vi "Position.vi"   [LabVIEW 2011]
uses:
  Robot Global Data.vi
types:
  T1 = typedef "WPI_EncoderDevRef.ctl" = cluster{"DevStatus":errorcluster, "EncoderIndex":T2, "CounterIndex":T3, "DistancePerCount":dbl, "Decoding Type":T4}
  T2 = typedef "FPGA_EncoderIdx.ctl" = enum8{"Enc 0", "Enc 1", "Enc 2", "Enc 3", "Invalid"}
  T3 = typedef "FPGA_CounterCtrSystemIndex.ctl" = enum8{"Ctr 0", "Ctr 1", "Ctr 2", "Ctr 3", "Ctr 4", "Ctr 5", "Ctr 6", "Ctr 7", "Invalid"}
  T4 = typedef "WPI_EncoderType.ctl" = enum16{"1x", "2x", "4x"}
  T5 = typedef "WPI_GyroDevRef.ctl" = cluster{"DevStatus":errorcluster, "Analog Module":T6, "Analog Channel":T7, "Offset":dbl, "Gain (VoltsPerDegree/Second)":dbl}
  T6 = typedef "FPGA_TypedefAnalogModule.ctl" = enum16{"Analog Module 1", "Analog Module 2"}
  T7 = typedef "FPGA_AIChannel.ctl" = enum8{"AI 1", "AI 2", "AI 3", "AI 4", "AI 5", "AI 6", "AI 7", "AI 8", "Invalid"}
  T8 = typedef "Position Typedef.ctl" = cluster{"X":dbl, "Y":dbl, "Heading":dbl}
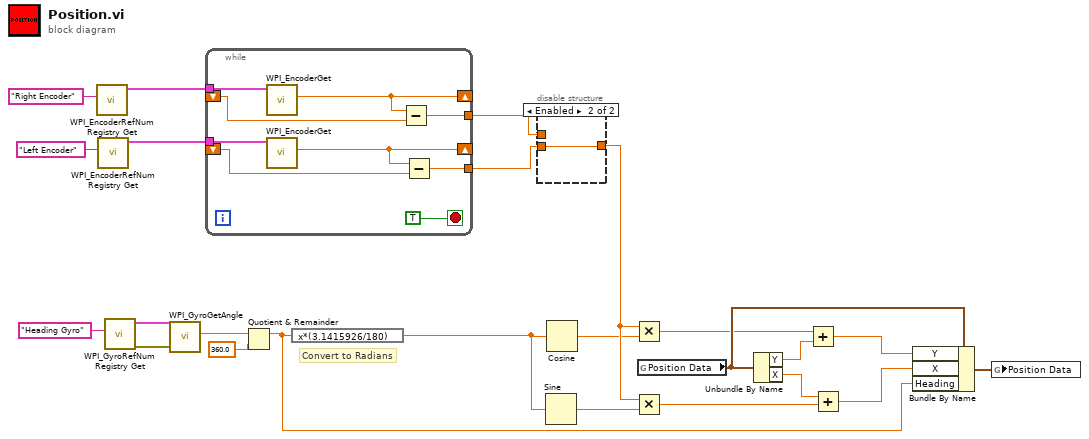
[diagram p0: block diagram]
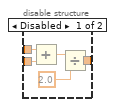
[diagram p2: hidden frame]
diagram:
  # "Convert to Radians"
  n1 = call <vilib>:"WPI_EncoderRefNum Registry Get.vi"("refnum name"="Right Encoder") -> ("EncoderDevRef"=w4:T1)  [unwired: 1 in, 9 out]
  n2 = call <vilib>:"WPI_EncoderRefNum Registry Get.vi"("refnum name"="Left Encoder") -> ("EncoderDevRef"=w5:T1)  [unwired: 1 in, 9 out]
  n3 = call <vilib>:"WPI_GyroRefNum Registry Get.vi"("refnum name"="Heading Gyro") -> ("error out"=w12:errorcluster, "GyroDevRef"=w11:T5)  [unwired: 1 in, 8 out]
  n4 = call <vilib>:"WPI_GyroGetAngle.vi"("error in (no error)"=w12, "GyroDevRef"=w11) -> ("Angle"=w8:dbl)  [unwired: 9 out]
  n5 = while {
    tunnel: w4 -> [w33]
    tunnel: w5 -> [w32]
    shift-right: [w31] -> _
    shift-left: _ -> [w30]
    shift-right: [w29] -> _
    shift-left: _ -> [w28]
    tunnel: [w27] -> w6
    tunnel: [w26] -> w7
    stop <- TRUE stop-if-true
    n6 = call <vilib>:"WPI_EncoderGet.vi"("EncoderDevRef"=w33) -> ("Distance"=w31:dbl)  [unwired: 1 in, 9 out]
    n7 = call <vilib>:"WPI_EncoderGet.vi"("EncoderDevRef"=w32) -> ("Distance"=w29:dbl)  [unwired: 1 in, 9 out]
    n8 = Subtract(x=w31, y=w30) -> (x-y=w27:dbl)
    n9 = Subtract(x=w29, y=w28) -> (x-y=w26:dbl)
  }
  n10 = Quotient & Remainder(x=w8, y=360.0) -> (x-y*floor(x/y)=w24:dbl)  [unwired: 1 out]
  n11 = expression code="x*(3.1415926/180)"(w24) -> (w10:dbl)
  n12 = disable-structure shown="Enabled" {
    disable-tunnel: [w38 w39] -> w14
    disable-tunnel: w7 -> [w37 w39]
    disable-tunnel: w6 -> [w36 _]
    frame Disabled {
      n13 = Add(x=w36, y=w37) -> (x+y=w34:dbl)
      n14 = Divide(x=w34, y=2.0) -> (x/y=w38:dbl)
    }
    frame Enabled {
    }
  }
  n15 = Sine(x=w10) -> (sin(x)=w15:dbl)
  n16 = Cosine(x=w10) -> (cos(x)=w13:dbl)
  n17 = Multiply(x=w14, y=w13) -> (x*y=w16:dbl)
  n18 = Multiply(x=w14, y=w15) -> (x*y=w18:dbl)
  n19 = global read "Robot Global Data.vi" "Position Data"() -> (w21:T8)
  n20 = Unbundle By Name(w21) -> ("Y"=w17:dbl, "X"=w19:dbl)
  n21 = Add(x=w16, y=w17) -> (x+y=w22:dbl)
  n22 = Add(x=w19, y=w18) -> (x+y=w23:dbl)
  n23 = Bundle By Name(cluster=w21, "Y"=w22, "X"=w23, "Heading"=w24) -> (w20:T8)
  n24 = global write "Robot Global Data.vi" "Position Data"(w20) -> ()
